vi "Read Color.vi"(8 "error in (no error)":errorcluster, 11 "DrawComponent in":refnum<class "DrawComponent.lvclass">) -> (0 "error out":errorcluster, 2 "Color":u32(colorbox), 3 "DrawComponent out":refnum<class "DrawComponent.lvclass">)   [LabVIEW 2022 SP3, in "DrawComponent.lvclass"]
uses:
  DrawComponent.lvclass
  DrawComponent.lvclass/DrawComponent.ctl
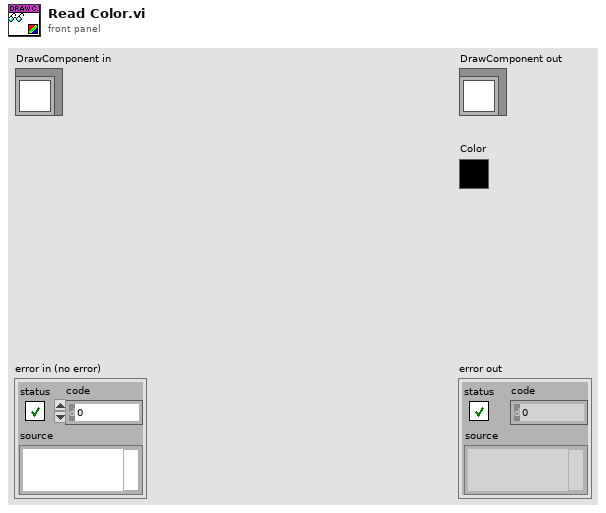
[diagram p1: front panel]
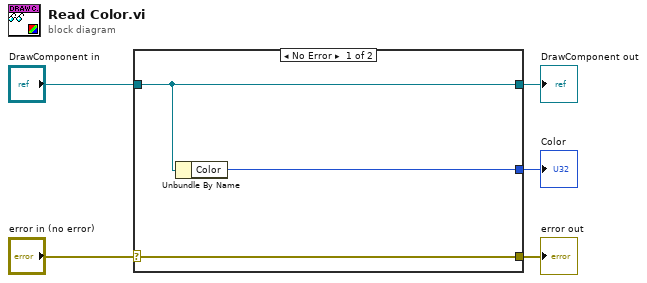
[diagram p0: block diagram]
diagram:
  n1 = case shown="No Error" "error in (no error)" {
    selector: "error in (no error)" -> [w8 w9]
    tunnel: [w8 w9] -> w4
    tunnel: [w7 w10] -> w2
    tunnel: "DrawComponent in" -> [w7 w10]
    tunnel: [w6 _] -> w1
    frame No Error {
      n2 = Unbundle By Name(w7) -> ("Color"=w6:u32)
    }
    frame Error {
    }
  }
  "error out" <- w4
  "DrawComponent out" <- w2
  "Color" <- w1
